vi "BufferUnescape.vi"(9 "XOR Byte":u8=32, 10 "EscapeByte":u8=125, 11 "Buffer In":u8[](array[numeric])) -> (3 "Buffer Out":u8[](array[numeric]))   [LabVIEW 2009]
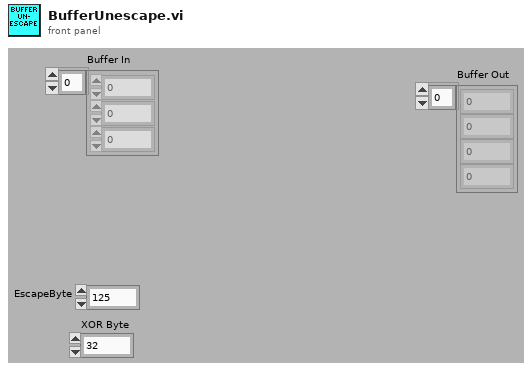
[diagram p1: front panel]
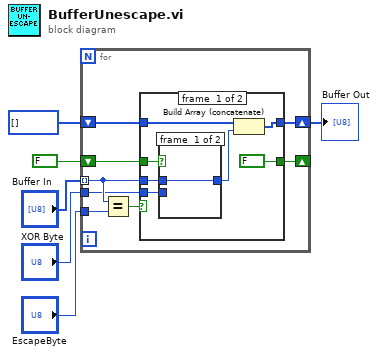
[diagram p0: block diagram]
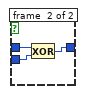
[diagram p2: hidden frame]
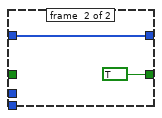
[diagram p3: hidden frame]
diagram:
  n1 = for {
    tunnel: "Buffer In" -> [w10] mode=indexing
    shift-right: [w8] -> w4
    shift-left: u8[] [] -> [w9]
    shift-right: [w12] -> _
    shift-left: FALSE -> [w11]
    tunnel: "EscapeByte" -> [w14]
    tunnel: "XOR Byte" -> [w7]
    n2 = Equal?(x=w10, y=w14) -> (x = y?=w13:bool)
    n3 = case shown="False" w13 {
      tunnel: [FALSE TRUE] -> w12
      tunnel: w11 -> [w20 _]
      tunnel: w10 -> [w19 _]
      tunnel: w9 -> [w18 w26]
      tunnel: [w17 w26] -> w8
      tunnel: w7 -> [w15 _]
      frame #0 {
        n4 = case shown="True" w20 {
          tunnel: w19 -> [w22 w25]
          tunnel: [w22 w23] -> w16
          tunnel: w15 -> [_ w24]
          frame #0 {
          }
          frame #1 {
            n5 = Exclusive Or(1:w24, 2:w25) -> (0:w23:u8)
          }
        }
        n6 = Build Array (concatenate)(w18, w16) -> (w17:u8[])
      }
      frame #1 {
      }
    }
  }
  "Buffer Out" <- w4
